vi "User-Defined IO Variable - Basic (Host).vi"() -> ()   [LabVIEW 2015]
doc: "This VI shows how to pass values from the host to the FPGA and back from the FPGA to the host using the user-defined I/O variable. It also shows how to use user-defined I/O variable scaling."
uses:
  <vilib>/rvi/interface/nirviOpenFPGA/nirviOpenFPGA.xnode
  <vilib>/rvi/interface/nirviCloseFPGA/nirviCloseFPGA.xnode
  <vilib>/rvi/interface/nirviMethod/nirviMethod.xnode
  <vilib>/rvi/errors/niLvFpgaMergeErrorWithErrorCode.vi
  FPGA Bitfiles/User-DefinedIOVa_FPGATarget2_User-DefinedIOVa_-uHZtoRN-no.lvbitx
  User-Defined IO Variable - Basic.vi
panel:
  out "error out":errorcluster
  in  "Host to FPGA: Boolean":bool
  in  "Stop":bool
  in  "Host to FPGA: Integer":u32
  out "FPGA to Host: Boolean":bool
  out "FPGA to Host: Integer":u32
  # "Overview: Demonstrates how to pass values to and from the FPGA through user-defined I/O variables. Refer to the Transferring Data Between the FPGA and Host VI (FPGA Module) topic of the LabVIEW Help for more information.\nRequirements: LabVIEW Real-Time Module, LabVIEW FPGA Module, NI-RIO\nInstructions: \n1. Compile the FPGA VI\n2. Run the VI.\n3. Enter a value, from 0-10, in the Host to FPGA: Integer control. The FPGA to Host: Integer indicator will return the value scaled to a range of 0-100. The scaling can be configured in the User-Defined I/O Variable properties page, accessible from the project.\n4. Click Stop to stop the VI."
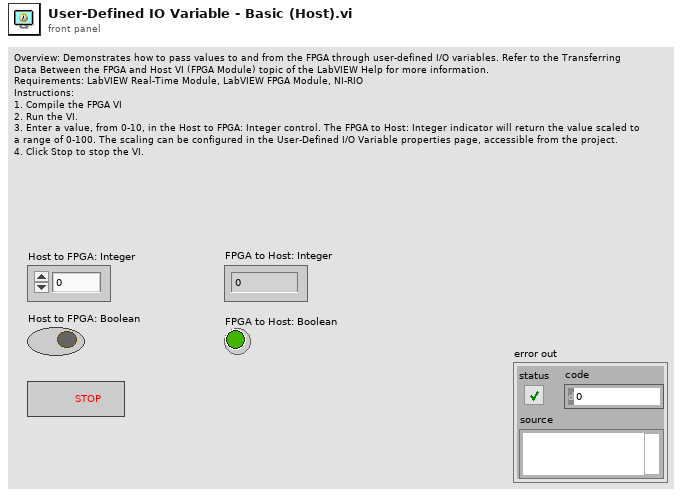
[diagram p1: front panel]
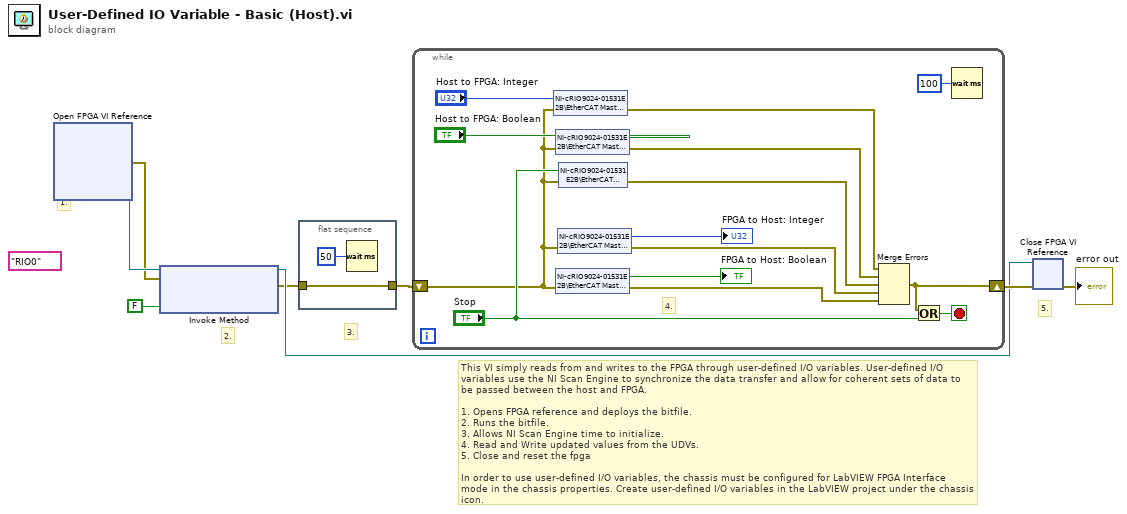
[diagram p0: block diagram]
diagram:
  (unwired) tag "RIO0" ("resource name")
  # "5."
  # "3."
  # "2."
  # "1."
  # "This VI simply reads from and writes to the FPGA through user-defined I/O variables. User-defined I/O variables use the NI Scan Engine to synchronize the data transfer and allow for coherent sets of data to be passed between the host and FPGA. \n\n1. Opens FPGA reference and deploys the bitfile.\n2. Runs the bitfile.\n3. Allows NI Scan Engine time to initialize.\n4. Read and Write updated values from the UDVs. \n5. Close and reset the fpga\n\nIn order to use user-defined I/O variables, the chassis must be configured for LabVIEW FPGA Interface mode in the chassis properties. Create user-defined I/O variables in the LabVIEW project under the chassis icon."
  n1 = xnode "Open FPGA VI Reference"() -> ("FPGA VI Reference Out"=w6:refnum<k20>, "error out"=w1:errorcluster)  [unwired: 2 in]
  n2 = xnode "Invoke Method"("FPGA VI Reference In"=w6, "error in"=w1, "Wait Until Done (F)"=FALSE) -> ("FPGA VI Reference Out"=w5:refnum<k20>, "error out"=w3:errorcluster)
  n3 = flat-sequence {
    tunnel: w3 -> [w9]
    tunnel: [w9] -> w2
    frame #0 {
      n4 = Wait (ms)(milliseconds to wait=u32 50) -> ()  [unwired: 1 out]
    }
  }
  n5 = while {
    shift-right: [w17] -> w7
    shift-left: w2 -> [w12]
    stop <- w23 stop-if-true
    # "4."
    n6 = shared-variable "NI-cRIO9024-01531E2B\\EtherCAT Master\\Device\\User-Defined Variables\\HFInt"("Host to FPGA: Integer", error in=w12) -> (error out=w13:errorcluster)
    n7 = shared-variable "NI-cRIO9024-01531E2B\\EtherCAT Master\\Device\\User-Defined Variables\\HFBo"("Host to FPGA: Boolean", error in=w12) -> (error out=w14:errorcluster)
    n8 = shared-variable "NI-cRIO9024-01531E2B\\EtherCAT Master\\Device\\User-Defined Variables\\FHBo"(error in=w12) -> (→"FPGA to Host: Boolean":bool, error out=w16:errorcluster)
    n9 = shared-variable "NI-cRIO9024-01531E2B\\EtherCAT Master\\Device\\User-Defined Variables\\FHInt"(error in=w12) -> (→"FPGA to Host: Integer":i32, error out=w11:errorcluster)
    n10 = shared-variable "NI-cRIO9024-01531E2B\\EtherCAT Master\\Device\\User-Defined Variables\\Stop"("Stop", error in=w12) -> (error out=w15:errorcluster)
    n11 = Merge Errors(w13, w14, w15, w11, w16) -> (w17:errorcluster)
    n12 = Or(x=w17, y="Stop") -> (x .or. y?=w23:bool)
    n13 = Wait (ms)(milliseconds to wait=u32 100) -> ()  [unwired: 1 out]
  }
  n14 = xnode "Close FPGA VI Reference"("FPGA VI Reference In"=w5, "error in"=w7) -> ("error out"=→"error out":errorcluster)
